vi "channel add.vi"(10 "number of channels (1)":i32=1) -> (0 "error out":errorcluster, 1 "lines match?":bool, 2 "channels":refnum<class "TBM channel.lvclass">[](array[class]), 3 "configuration out":refnum<class "Shared Memory Configuration.lvclass">, 4 "valid?":bool)   [LabVIEW 2013, in "Shared Memory Tests.lvlib"]
uses:
  Shared Memory Tests.lvlib
  module/configuration/Shared Memory Configuration.lvclass
  <vilib>/NI/Tag Bus Module Framework/channel/TBM channel.lvclass
  <vilib>/NI/Tag Bus Module Framework/channel/channel classification.ctl
  module/configuration/Shared Memory Configuration.lvclass/Shared Memory Configuration.ctl
  <vilib>/NI/Tag Bus/tag/tag descriptor.lvclass/tag descriptor.ctl
  module/configuration/Write Read Directory.vi
  module/configuration/Write Write Directory.vi
  <vilib>/NI/Configuration Framework/serializable configuration/NISE_CEF_serializable configuration.lvclass
  <vilib>/NI/Tag Bus/tag/tag descriptor.lvclass
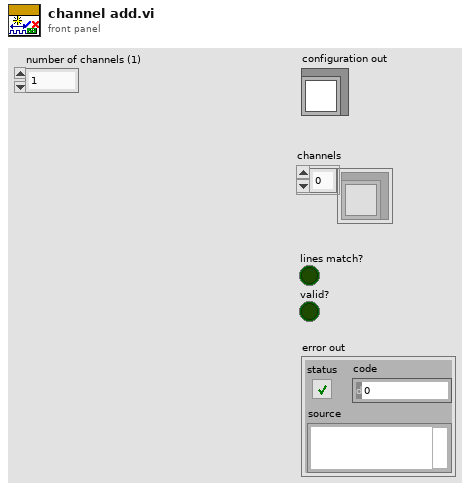
[diagram p1: front panel]
types:
  T1 = typedef "TBM channel.lvclass/channel classification.ctl" = enum16{"input data", "output data", "processing parameter", "processing result"}
  T2 = typedef "tag bus.lvlib/tag descriptor.lvclass/Data Type.ctl" = enum16{"Double", "Single", "I64", "I32", "I16", "I8", "U64", "U32", "U16", "U8", "Boolean", "String", "Array of Double", "Array of Single", "Array of I64", "Array of I32", "Array of I16", "Array of I8", "Array of U64", "Array of U32", "Array of U16", "Array of U8", "Array of Boolean", "Array of String"}
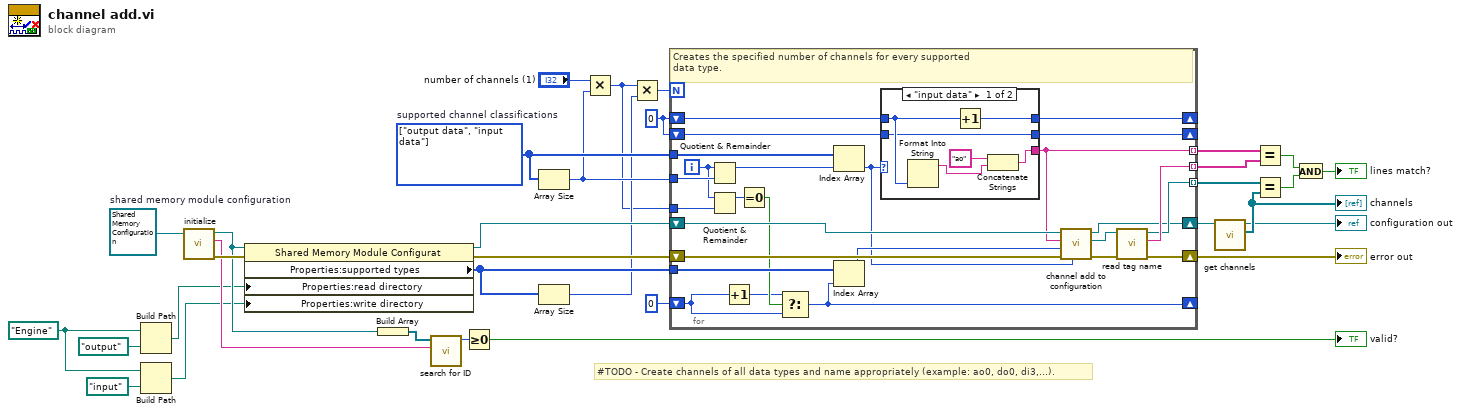
[diagram p0: block diagram]
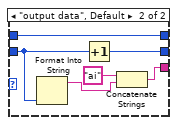
[diagram p2: hidden frame]
diagram:
  w8 = T1[] [enum."output data", enum."input data"] items=["input data", "output data", "processing parameter", "processing result"]  # supported channel classifications
  w11 = 0
  w1 = path "Engine"
  w30 = refnum<class "Shared Memory Configuration.lvclass"> refnum  # shared memory module configuration
  # "#TODO - Create channels of all data types and name appropriately (example: ao0, do0, di3,...)."
  n1 = Build Path(base path=w1, name or relative path=path "output") -> (appended path=w13:path)
  n2 = Build Path(base path=w1, name or relative path=path "input") -> (appended path=w12:path)
  n3 = call <vilib>:"initialize.vi"("configuration in"=w30) -> ("error out"=w33:errorcluster, "identifier"=w22:string, "configuration out"=w24:refnum<class "Shared Memory Configuration.lvclass">)  [unwired: 8 in]
  n4 = property class="Shared Memory Module Configurat"(reference=w24, error in=w33, "Properties:read directory"=w13, "Properties:write directory"=w12) -> (reference out=w31:refnum<class "Shared Memory Configuration.lvclass">, error out=w32:errorcluster, "Properties:supported types"=w10:T2[])
  n5 = Build Array(w24) -> (w23:refnum<class "Shared Memory Configuration.lvclass">[])
  n6 = call <vilib>:"search for ID.vi"("instance id"=w22, "instance data"=w23) -> ("index"=w21:i32)  [unwired: 9 in]
  n7 = Greater Or Equal To 0?(x=w21) -> (x >= 0?=→"valid?":bool)
  n8 = Array Size(array=w8) -> (size(s)=w5:i32)
  n9 = Array Size(array=w10) -> (size(s)=w4:i32)
  n10 = Multiply(x="number of channels (1)", y=w5) -> (x*y=w2:i32)
  n11 = Multiply(x=w2, y=w4) -> (x*y=w3:i32)
  n12 = for {
    N: w3 -> [_]
    shift-right: [w52] -> w29
    shift-left: w31 -> [w58]
    shift-right: [w53] -> w9
    shift-left: w32 -> [w59]
    tunnel: w10 -> [w46]
    tunnel: [w54] -> w26 mode=indexing
    tunnel: [w55] -> w27 mode=indexing
    tunnel: [w47] -> w28 mode=indexing
    shift-right: [w49] -> _
    shift-left: w11 -> [w51]
    shift-right: [w48] -> _
    shift-left: w11 -> [w50]
    tunnel: w8 -> [w43]
    tunnel: w5 -> [w44]
    shift-right: [w36] -> _
    shift-left: 0 -> [w35]
    tunnel: w2 -> [w39]
    i -> [w40]
    # "Creates the specified number of channels for every supported\ndata type."
    n13 = Quotient & Remainder(x=w40, y=w44) -> (x-y*floor(x/y)=w42:i32)  [unwired: 1 out]
    n14 = Quotient & Remainder(x=w40, y=w39) -> (x-y*floor(x/y)=w38:i32)  [unwired: 1 out]
    n15 = Increment(x=w35) -> (x+1=w34:i32)
    n16 = Equal To 0?(x=w38) -> (x = 0?=w37:bool)
    n17 = Select(t=w34, s=w37, f=w35) -> (s? t:f=w36:i32)
    n18 = Index Array(array=w43, index=w42) -> (element=w41:T1)
    n19 = Index Array(array=w46, index=w36) -> (element=w45:T2)
    n20 = case shown="\"input data\"" w41 {
      tunnel: w51 -> [w65 w66]
      tunnel: w50 -> [w61 w68]
      tunnel: [w62 w66] -> w49
      tunnel: [w61 w67] -> w48
      tunnel: [w60 w69] -> w47
      frame "input data" {
        n21 = Format Into String(w65) -> (resulting string=w63:string)  [unwired: 3 in, 1 out]
        n22 = Increment(x=w65) -> (x+1=w62:i32)
        n23 = Concatenate Strings("ao", w63) -> (w60:string)
      }
      frame "output data", Default {
        n24 = Format Into String(w68) -> (resulting string=w70:string)  [unwired: 3 in, 1 out]
        n25 = Increment(x=w68) -> (x+1=w67:i32)
        n26 = Concatenate Strings("ai", w70) -> (w69:string)
      }
    }
    n27 = call "channel add to configuration.vi"("channel classification (output data)"=w41, "error in"=w59, "data type"=w45, "channel name"=w47, "shared memory module configuration in"=w58) -> ("error out"=w56:errorcluster, "created channel"=w57:refnum<class "TBM channel.lvclass">, "shared memory module configuration out"=w52:refnum<class "Shared Memory Configuration.lvclass">)  [unwired: 4 in]
    n28 = call <vilib>:"read tag name.vi"("error in"=w56, "system tag in"=w57) -> ("error out"=w53:errorcluster, "name"=w55:string, "system tag out"=w54:refnum<class "TBM channel.lvclass">)  [unwired: 7 in]
  }
  "error out" <- w9
  n29 = call-dynamic "get channels.vi"("shared memory module configuration"=w29) -> ("channels"=w25:refnum<class "TBM channel.lvclass">[], "shared memory module configuration out"=→"configuration out":refnum<class "Shared Memory Configuration.lvclass">)  [unwired: 9 in]
  "channels" <- w25
  n30 = Equal?(x=w28, y=w27) -> (x = y?=w18:bool)
  n31 = Equal?(x=w26, y=w25) -> (x = y?=w17:bool)
  n32 = And(x=w18, y=w17) -> (x .and. y?=→"lines match?":bool)
